vi "Drive PID.vi"(4 "reinitialize? (F)":bool, 5 "output range":T1={"output high"=1.0, "output low"=-1.0}, 6 "PID Params":T2={"PID gains"={"proportional gain (Kc)"=1.0, "integral time (Ti, min)"=0.0, "derivative time (Td, min)"=0.0}}, 7 "Setpoint":dbl, 8 "Max Stop Speed":dbl, 9 "Distance Stop Threshold":dbl, 10 "Current Speed":dbl, 11 "Current Distance":dbl format="%#_13g") -> (0 "Finished":bool, 2 "output":dbl format="%.2f")   [LabVIEW 2014]
uses:
  Drivetrain Output Range.ctl
  <vilib>/addons/control/pid/pid.llb/PID (DBL).vi
  <vilib>/addons/control/pid/NI_PID_pid.lvlib
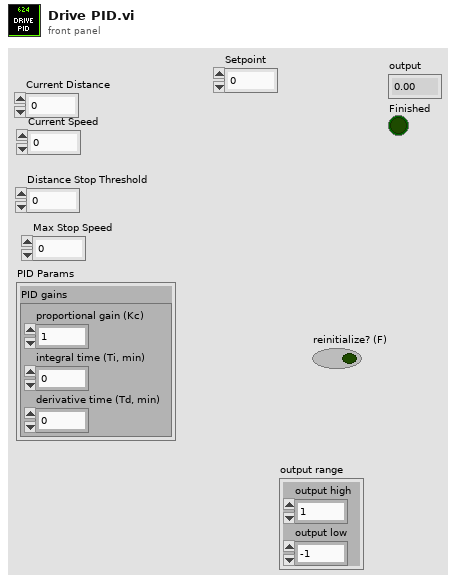
[diagram p1: front panel]
types:
  T1 = typedef "Drivetrain Output Range.ctl" = cluster{"output high":dbl, "output low":dbl}
  T2 = cluster{"PID gains":cluster{"proportional gain (Kc)":dbl, "integral time (Ti, min)":dbl, "derivative time (Td, min)":dbl}}
  T3 = cluster{"proportional gain (Kc)":dbl, "integral time (Ti, min)":dbl, "derivative time (Td, min)":dbl}
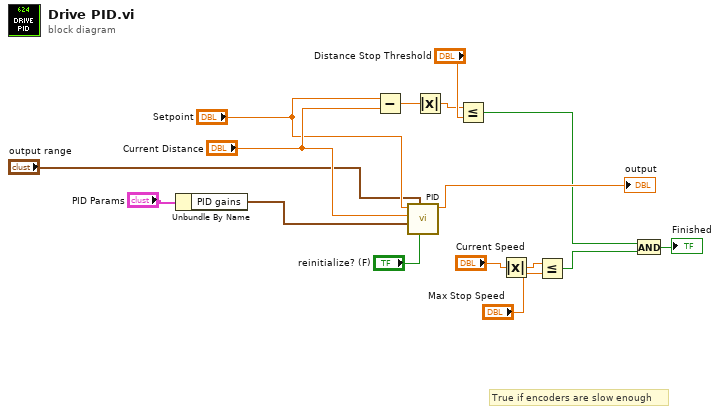
[diagram p0: block diagram]
diagram:
  # "True if encoders are slow enough"
  n1 = Unbundle By Name("PID Params") -> ("PID gains"=w13:T3)
  n2 = Subtract(x="Setpoint", y="Current Distance") -> (x-y=w10:dbl)
  n3 = call-poly <vilib>:"PID.vi"("reinitialize? (F)"="reinitialize? (F)", "output range"="output range", "PID gains"=w13, "process variable"="Current Distance", "setpoint"="Setpoint") -> ("output"=→"output":dbl)  [unwired: 5 in, 1 out]
  n4 = Absolute Value(x=w10) -> (abs(x)=w8:dbl)
  n5 = Less Or Equal?(x=w8, y="Distance Stop Threshold") -> (x <= y?=w7:bool)
  n6 = Absolute Value(x="Current Speed") -> (abs(x)=w2:dbl)
  n7 = Less Or Equal?(x=w2, y="Max Stop Speed") -> (x <= y?=w5:bool)
  n8 = And(x=w7, y=w5) -> (x .and. y?=→"Finished":bool)
